vi "3.2.vi"(1 "B":dbl, 2 "A":dbl, 3 "枚举":enum16{"相除", "相减", "相乘", "相加"}(ring)) -> (0 "Result":dbl)   [LabVIEW 2017]
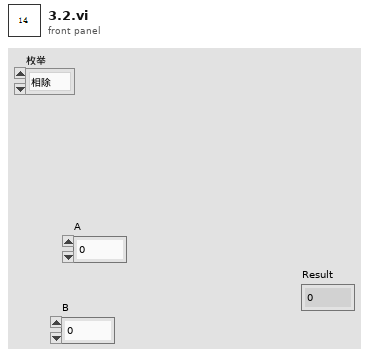
[diagram p1: front panel]
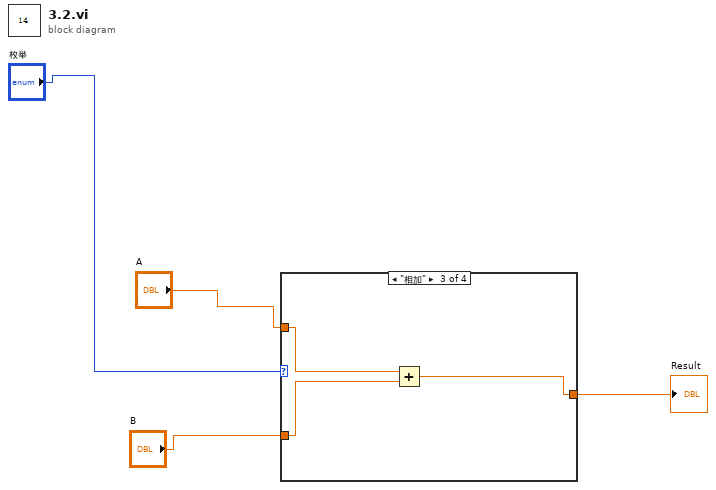
[diagram p0: block diagram]
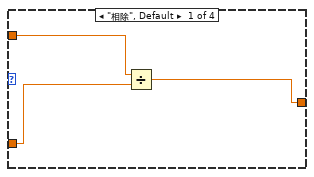
[diagram p2: hidden frame]
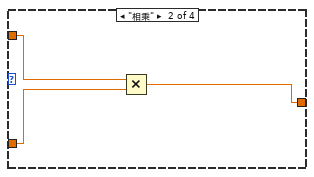
[diagram p3: hidden frame]
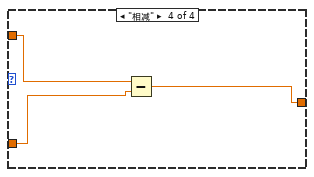
[diagram p4: hidden frame]
diagram:
  n1 = case shown="\"相加\"" "枚举" {
    tunnel: "A" -> [w7 w9 w12 w15]
    tunnel: "B" -> [w5 w8 w11 w14]
    tunnel: [w6 w10 w13 w16] -> w1
    frame "相除", Default {
      n2 = Divide(x=w7, y=w5) -> (x/y=w6:dbl)
    }
    frame "相乘" {
      n3 = Multiply(x=w9, y=w8) -> (x*y=w10:dbl)
    }
    frame "相加" {
      n4 = Add(x=w12, y=w11) -> (x+y=w13:dbl)
    }
    frame "相减" {
      n5 = Subtract(x=w15, y=w14) -> (x-y=w16:dbl)
    }
  }
  "Result" <- w1
